vi "Run Motion Profile V2.0 (Right).vi"(11 "PhoenixMotorControlDevRef In":T2={"DeviceStatus"={"status"=FALSE, "code"=0, "source"=""}, "Type"=enum."PWM", "PWM"={"PWM Channel"=enum."Invalid", "DeadBand"={"Name"="", "maxPositivePwm"=0, "minPositivePwm"=0, "centerPwm"=0, "maxNegativePwm"=0, "minNegativePwm"=0, "angularRange"=0}}, "CAN"={"Device Number"=0, "SetOutput VI Ref"=variant(enum8{"Percent VBus", "Current", "Speed", "Position", "Voltage"} enum."Percent VBus"), "GetOutput VI Ref"=variant(refnum<k1> refnum), "Enable VI Ref"=variant(dbl 12.0), "Disable VI Ref"=variant(enum8{"Percent VBus", "Speed", "Position", "Slave", "Unchanged / Invalid", "Voltage Compensation", "Current", "Motion Profile"} enum."Percent VBus"), "Data"=variant}, "Invert"=FALSE, "DIO PWM"={"PWM \"Enable\" Channel"=enum."Invalid", "DIOChannel"=enum."Invalid", "PWM Rate"=0.0}}) -> ()   [LabVIEW 2017]
uses:
  <vilib>/Rock Robotics/WPI/MotorControl/WPI_MotorControlDeviceRef.ctl
  <vilib>/Rock Robotics/WPI/MotorControl/WPI_MotorControlType.ctl
  <vilib>/Rock Robotics/SystemInterfaces/DIO/FPGA_DIOPWMChannel.ctl
  <vilib>/Rock Robotics/WPI/PWM/WPI_PWMDeadband.ctl
  <vilib>/Rock Robotics/SystemInterfaces/DIO/FPGA_DIOChannel.ctl
  TrajectoryPointClusterV2.0.ctl
  <vilib>/Rock Robotics/WPI/ThirdParty/Phoenix-LabVIEW/Motor Controller/Controls/CTRE_Phoenix_MotorControl_TrajectoryPointTimeDur.ctl
  Motion Profile Global Variable.vi
panel:
  out "Trajectory":T1[](array[typedef])
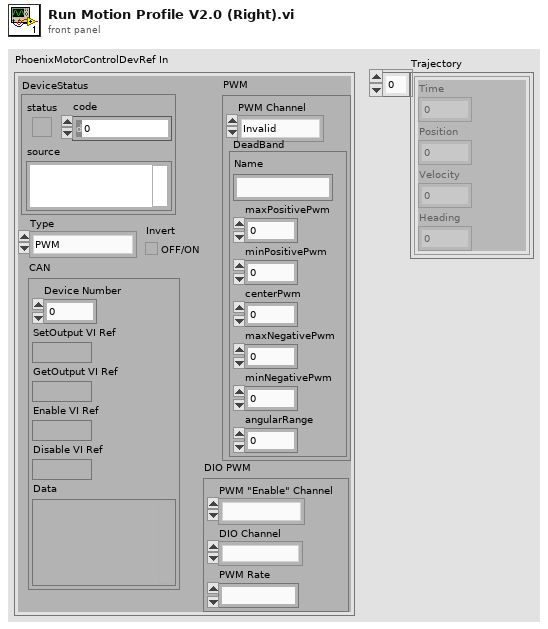
[diagram p1: front panel]
types:
  T1 = typedef "TrajectoryPointClusterV2.0.ctl" = cluster{"Position":dbl, "Velocity":dbl, "Heading":dbl, "Time":dbl}
  T2 = typedef "WPI_MotorControlDeviceRef.ctl" = cluster{"DeviceStatus":errorcluster, "Type":T3, "PWM":cluster{"PWM Channel":T4, "DeadBand":T5}, "CAN":cluster{"Device Number":u8, "SetOutput VI Ref":variant, "GetOutput VI Ref":variant, "Enable VI Ref":variant, "Disable VI Ref":variant, "Data":variant}, "Invert":bool, "DIO PWM":cluster{"PWM \"Enable\" Channel":T4, "DIOChannel":T6, "PWM Rate":dbl}}
  T3 = typedef "WPI_MotorControlType.ctl" = enum16{"PWM", "CAN", "DIO PWM"}
  T4 = typedef "FPGA_DIOPWMChannel.ctl" = enum8{"PWM 0", "PWM 1", "PWM 2", "PWM 3", "PWM 4", "PWM 5", "PWM 6", "PWM 7", "PWM 8", "PWM 9", "PWM MXP 0", "PWM MXP 1", "PWM MXP 2", "PWM MXP 3", "PWM MXP 4", "PWM MXP 5", "PWM MXP 6", "PWM MXP 7", "PWM MXP 8", "PWM MXP 9", "Invalid"}
  T5 = typedef "WPI_PWMDeadband.ctl" = cluster{"Name":string, "maxPositivePwm":i32, "minPositivePwm":i32, "centerPwm":i32, "maxNegativePwm":i32, "minNegativePwm":i32, "angularRange":u16}
  T6 = typedef "FPGA_DIOChannel.ctl" = enum8{"DIO 0", "DIO 1", "DIO 2", "DIO 3", "DIO 4", "DIO 5", "DIO 6", "DIO 7", "DIO 8", "DIO 9", "DIO MXP 0", "DIO MXP 1", "DIO MXP 2", "DIO MXP 3", "DIO MXP 4", "DIO MXP 5", "DIO MXP 6", "DIO MXP 7", "DIO MXP 8", "DIO MXP 9", "DIO MXP 10", "DIO MXP 11", "DIO MXP 12", "DIO MXP 13", "DIO MXP 14", "DIO MXP 15", "SPI Port CS1", "SPI Port CS2", "SPI Port CS3", "SPI Port MISO", "SPI Port MOSI", "Invalid"}
  T7 = cluster{"Top Buffer Remaining":i32, "Top Buffer Count":i32, "Bottom Buffer Count":i32, "Has Underrun?":bool, "Is Underrun?":bool, "Active Point Valid?":bool, "Is Last?":bool, "Profile Slot Select 0":i32, "Output Enable":i32, "Time Duration (ms)":i32, "Profile Slot Select 1":i32}
  T8 = typedef "CTRE_Phoenix_MotorControl_TrajectoryPointTimeDur.ctl" = i32
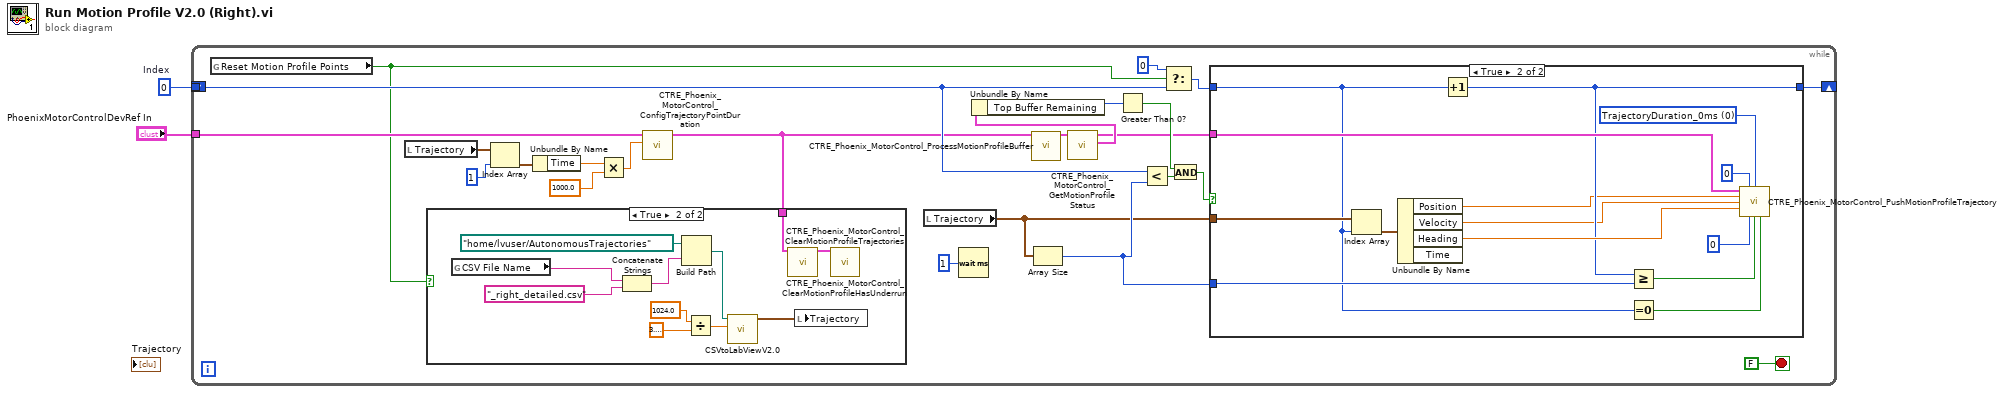
[diagram p0: block diagram]
diagram:
  w2 = 0  # Index
  n1 = while {
    shift-right: [w24] -> _
    shift-left: w2 -> [w19]
    tunnel: w2 -> [_]
    tunnel: "PhoenixMotorControlDevRef In" -> [w11]
    stop <- FALSE stop-if-true
    n2 = global read "Motion Profile Global Variable.vi" "Reset Motion Profile Points"() -> (w3:bool)
    n3 = local read "Trajectory"() -> (w9:T1[])
    n4 = Index Array(array=w9, index=1) -> (element=w12:T1)
    n5 = Unbundle By Name(w12) -> ("Time"=w8:dbl)
    n6 = Multiply(x=w8, y=1000.0) -> (x*y=w6:dbl)
    n7 = call <vilib>:"CTRE_Phoenix_MotorControl_ConfigTrajectoryPointDuration.vi"("durationMs"=w6, "PhoenixMotorControlDevRef"=w11) -> ("PhoenixMotorControlDevRef"=w4:T2)  [unwired: 8 in, 1 out]
    n8 = case shown="True" w3 {
      tunnel: w4 -> [_ w28]
      frame False {
      }
      frame True {
        n9 = global read "Motion Profile Global Variable.vi" "CSV File Name"() -> (w27:string)
        n10 = Concatenate Strings(w27, "_right_detailed.csv") -> (w33:string)
        n11 = Build Path(base path=path "/home/lvuser/AutonomousTrajectories", name or relative path=w33) -> (appended path=w31:path)
        n12 = Divide(x=1024.0, y=3.141592653589793) -> (x/y=w32:dbl)
        n13 = call "CSVtoLabViewV2.0.vi"("Sensor Unit Conversion"=w32, "file path (dialog if empty)"=w31) -> ("Trajectory Point Array"=w30:T1[])  [unwired: 9 in]
        n14 = call <vilib>:"CTRE_Phoenix_MotorControl_ClearMotionProfileTrajectories.vi"("PhoenixMotorControlDevRef"=w28) -> ("PhoenixMotorControlDevRef"=w29:T2)  [unwired: 13 in, 1 out]
        n15 = local write "Trajectory"(w30) -> ()
        n16 = call <vilib>:"CTRE_Phoenix_MotorControl_ClearMotionProfileHasUnderrun.vi"("PhoenixMotorControlDevRef"=w29) -> ()  [unwired: 9 in, 2 out]
      }
    }
    n17 = local read "Trajectory"() -> (w5:T1[])
    n18 = Wait (ms)(milliseconds to wait=u32 1) -> ()  [unwired: 1 out]
    n19 = call <vilib>:"CTRE_Phoenix_MotorControl_ProcessMotionProfileBuffer.vi"("PhoenixMotorControlDevRef"=w4) -> ("PhoenixMotorControlDevRef"=w20:T2)  [unwired: 13 in, 1 out]
    n20 = Array Size(array=w5) -> (size(s)=w18:i32)
    n21 = call <vilib>:"CTRE_Phoenix_MotorControl_GetMotionProfileStatus.vi"("PhoenixMotorControlDevRef"=w20) -> ("Motion Profile Status"=w21:T7, "PhoenixMotorControlDevRef"=w10:T2)  [unwired: 8 in, 1 out]
    n22 = Unbundle By Name(w21) -> ("Top Buffer Remaining"=w17:i32)
    n23 = Greater Than 0?(x=w17) -> (x > 0?=w16:bool)
    n24 = Less?(x=w19, y=w18) -> (x < y?=w26:bool)
    n25 = Select(t=0, s=w3, f=w19) -> (s? t:f=w15:i32)
    n26 = And(x=w16, y=w26) -> (x .and. y?=w25:bool)
    n27 = case shown="True" w25 {
      tunnel: w5 -> [_ w52]
      tunnel: w10 -> [_ w49]
      tunnel: w18 -> [_ w47]
      tunnel: [w38 w42] -> w24
      tunnel: w15 -> [w38 w39]
      frame False {
      }
      frame True {
        w43 = T8 0 items=["TrajectoryDuration_0ms"=0, "TrajectoryDuration_5ms"=5, "TrajectoryDuration_10ms"=10, "TrajectoryDuration_20ms"=20, "TrajectoryDuration_30ms"=30, "TrajectoryDuration_40ms"=40, "TrajectoryDuration_50ms"=50, "TrajectoryDuration_100ms"=100] ("durationMs")
        n28 = Index Array(array=w52, index=w39) -> (element=w51:T1)
        n29 = Unbundle By Name(w51) -> ("Position"=w41:dbl, "Velocity"=w40:dbl, "Heading"=w50:dbl)  [unwired: 1 out]
        n30 = Increment(x=w39) -> (x+1=w42:i32)
        n31 = Greater Or Equal?(x=w42, y=w47) -> (x >= y?=w46:bool)
        n32 = Equal To 0?(x=w39) -> (x = 0?=w48:bool)
        n33 = call <vilib>:"CTRE_Phoenix_MotorControl_PushMotionProfileTrajectory.vi"("PhoenixMotorControlDevRef"=w49, "profileSlotSelect1"=0, "durationMs"=w43, "position"=w41, "velocity"=w40, "auxiliaryPos"=w50, "profileSlotSelect0"=0, "isLastPoint?"=w46, "Zero Position?"=w48) -> ()  [unwired: 5 in, 2 out]
      }
    }
  }
